vi "Initial Gen Cal.vi"(10 "Input String":string) -> (2 "Output String":string)   [LabVIEW 2010]
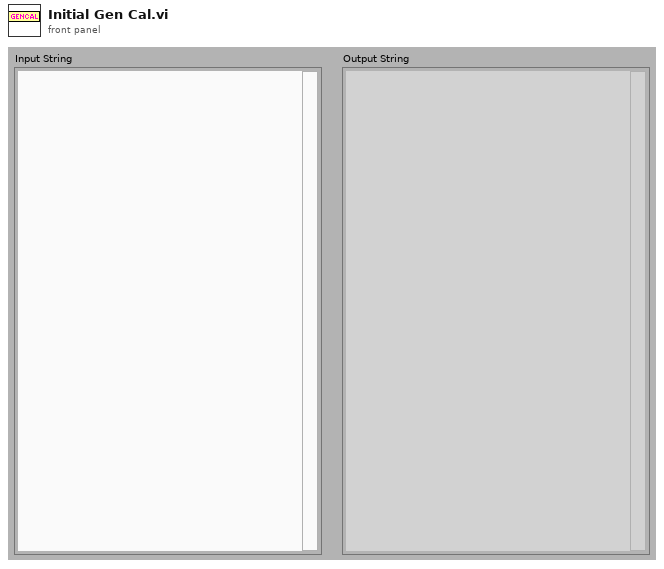
[diagram p1: front panel]
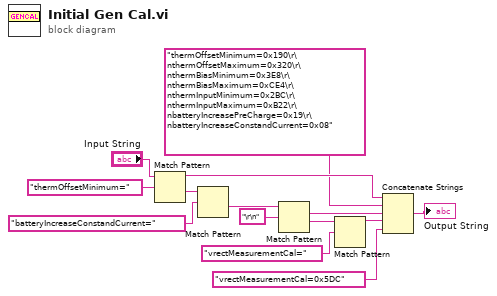
[diagram p0: block diagram]
diagram:
  n1 = Match Pattern(string="Input String", regular expression="thermOffsetMinimum=") -> (before substring=w12:string, after substring=w11:string)  [unwired: 1 in, 2 out]
  n2 = Match Pattern(string=w11, regular expression="batteryIncreaseConstandCurrent=") -> (after substring=w9:string)  [unwired: 1 in, 3 out]
  n3 = Match Pattern(string=w9, regular expression="\r\n") -> (match substring=w6:string, after substring=w4:string)  [unwired: 1 in, 2 out]
  n4 = Match Pattern(string=w4, regular expression="vrectMeasurementCal=") -> (before substring=w2:string)  [unwired: 1 in, 3 out]
  n5 = Concatenate Strings(w12, "thermOffsetMinimum=0x190\r\nthermOffsetMaximum=0x320\r\nthermBiasMinimum=0x3E8\r\nthermBiasMaximum=0xCE4\r\nthermInputMinimum=0x2BC\r\nthermInputMaximum=0xB22\r\nbatteryIncreasePreCharge=0x19\r\nbatteryIncreaseConstandCurrent=0x08" ("string"), w6, w2, "vrectMeasurementCal=0x5DC" ("regular expression")) -> (→"Output String":string)
